vi "UTEX Send Values MultiTry.vi"(5 "UT340 Controls":T1 {"Low Pass Filter (MHz)" min=20 step=1; "High Pass Filter (MHz)" min=1 max=20 step=1; "Pulse Width (ns)" min=2.0 max=71.75; "Voltage" min=100 max=250 step=2; "PC Gain (dB)" min=0 max=63 step=1; "PE Gain (dB)" min=-6 max=57 step=1}) -> (0 "Success":bool, 2 "UT340 Controls Out":T1={"High Pass On"=FALSE, "High Pass Filter (MHz)"=1, "Low Pass On"=FALSE, "Low Pass Filter (MHz)"=20, "PE Gain (dB)"=1, "Voltage"=100, "Pulse Width (ns)"=2.0, "Mode"=FALSE, "PC Gain (dB)"=1, "Trig Source"=FALSE, "Rep Rate (Hz)"=0, "PULSE"=FALSE} {"Low Pass Filter (MHz)" min=20 step=1; "High Pass Filter (MHz)" min=1 max=20 step=1; "Pulse Width (ns)" min=2.0 max=71.75; "Voltage" min=100 max=250 step=2; "PC Gain (dB)" min=0 max=63 step=1; "PE Gain (dB)" min=-6 max=57 step=1})   [LabVIEW 2022 SP3]
uses:
  Controls/UTEX Controls.ctl
  PulserGlobals.vi
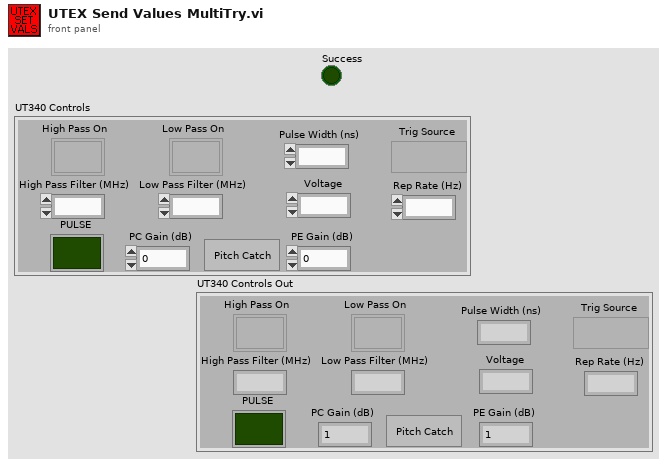
[diagram p1: front panel]
types:
  T1 = typedef "UTEX Controls.ctl" = cluster{"High Pass On":bool, "High Pass Filter (MHz)":i16, "Low Pass On":bool, "Low Pass Filter (MHz)":i16, "PE Gain (dB)":i16, "Voltage":i16, "Pulse Width (ns)":dbl, "Mode":bool, "PC Gain (dB)":i16, "Trig Source":bool, "Rep Rate (Hz)":i16, "PULSE":bool}
  T2 = cluster{"High Pass On":bool, "High Pass Filter (MHz)":bool, "Low Pass On":bool, "Low Pass Filter (MHz)":bool, "PE Gain (dB)":bool, "Voltage":bool, "Pulse Width (ns)":bool, "Mode":bool, "PC Gain (dB)":bool, "Trig Source":bool, "Rep Rate (Hz)":bool, "PULSE":bool}
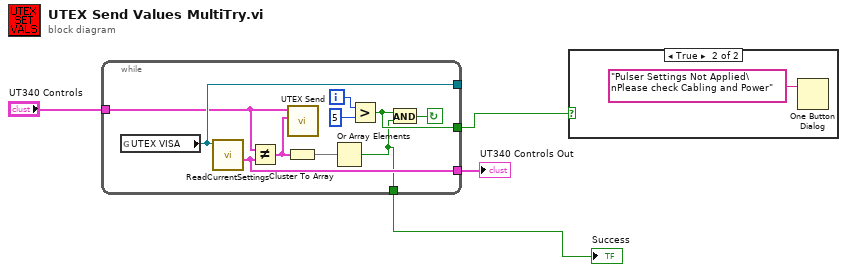
[diagram p0: block diagram]
diagram:
  n1 = while {
    tunnel: [w9] -> _
    tunnel: "UT340 Controls" -> [w8]
    tunnel: [w7] -> w3
    tunnel: [w6] -> w2
    tunnel: [w5] -> w1
    i -> [w12]
    stop <- w10 continue-if-true
    n2 = global read "PulserGlobals.vi" "UTEX VISA"() -> (w9:refnum<visa-resource-name>)
    n3 = call "ReadCurrentSettings.vi"("VISA Refnum in"=w9) -> ("UT340 Controls"=w7:T1)  [unwired: 8 in, 2 out]
    n4 = Not Equal?(x=w8, y=w7) -> (x != y?=w14:T2)
    n5 = Cluster To Array(cluster=w14) -> (array=w13:bool[])
    n6 = call "UTEX Send.vi"("Changed Values?"=w14, "UT340 Controls"=w8) -> ()  [unwired: 9 in, 1 out]
    n7 = Or Array Elements(Boolean array=w13) -> (logical OR=w5:bool)
    n8 = Greater?(x=w12, y=5) -> (0:w6:bool)
    n9 = And(x=w6, y=w5) -> (x .and. y?=w10:bool)
  }
  "UT340 Controls Out" <- w3
  "Success" <- w1
  n10 = case shown="True" w2 {
    frame False {
    }
    frame True {
      n11 = One Button Dialog(message="Pulser Settings Not Applied\nPlease check Cabling and Power") -> ()  [unwired: 1 in, 1 out]
    }
  }
